vi "Get Pin Access.vi"(4 "Signature Method":T1=enum."HMAC-SHA1", 5 "Consumer Secret":string, 6 "Use External Browser? (F)":bool, 7 "Consumer Key":string, 8 "error in (no error)":errorcluster, 9 "Access URL":string, 10 "Authorize URL":string, 11 "Request URL":string) -> (0 "error out":errorcluster, 1 "OAuth Credentials":T2={"Consumer Key"="", "Signature Method"=enum."HMAC-SHA1", "Token"="", "Version"="", "Token Secret"="", "Consumer Secret"=""}, 2 "body":string, 3 "headers":string)   [LabVIEW 2011, in "i3-oauth.lvlib"]
doc: "Obtains OAuth Credentials via PIN authorization for the application specified by the <B>Consumer Key</B> and <B>Consumer Secret</B>"
uses:
  i3-oauth.lvlib
  Controls/OAuth Credentials.ctl
  Controls/Signature Method.ctl
panel:
  in  "Callback URL":string="oob"
  # "For pin access, the callback URL is always oob"
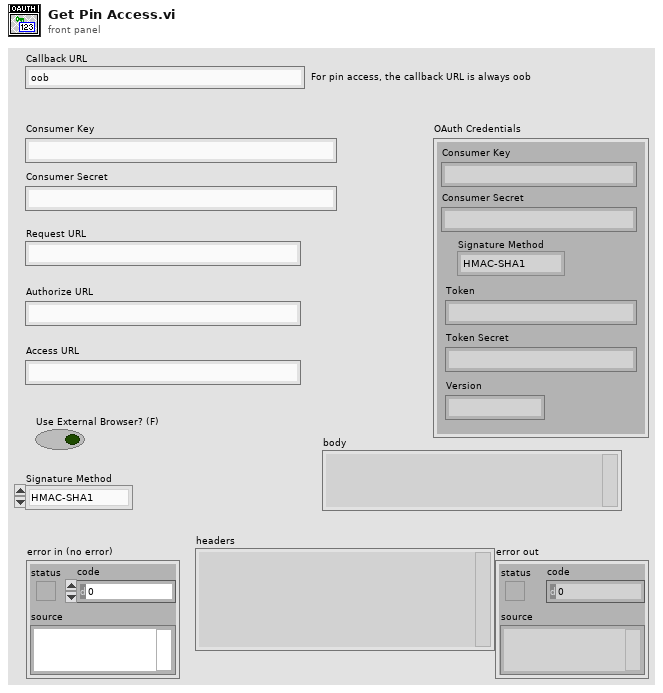
[diagram p1: front panel]
types:
  T1 = typedef "i3-oauth.lvlib/Signature Method.ctl" = enum16{"HMAC-MD5", "HMAC-SHA1", "HMAC-SHA224", "HMAC-SHA256", "HMAC-SHA384", "HMAC-SHA512"}
  T2 = typedef "i3-oauth.lvlib/OAuth Credentials.ctl" = cluster{"Consumer Key":string, "Signature Method":T1, "Token":string, "Version":string, "Token Secret":string, "Consumer Secret":string}
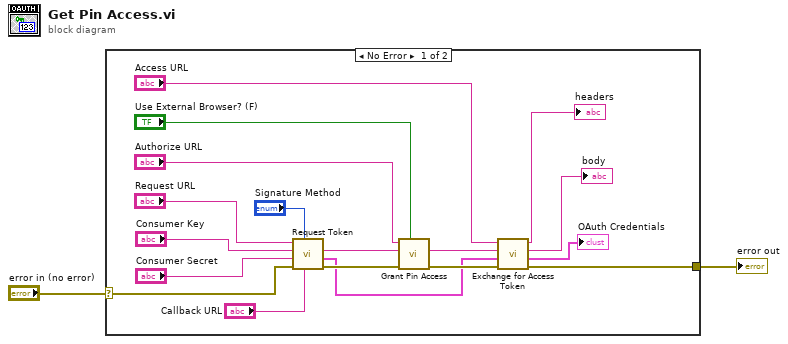
[diagram p0: block diagram]
diagram:
  n1 = case shown="No Error" "error in (no error)" {
    selector: "error in (no error)" -> [w11 w21]
    tunnel: [w10 w21] -> w1
    frame No Error {
      n2 = call "Request Token.vi"("Callback URL"="Callback URL", "Signature Method"="Signature Method", "error in (no error)"=w11, "Consumer Secret"="Consumer Secret", "Consumer Key"="Consumer Key", "Request URL"="Request URL") -> ("error out"=w20:errorcluster, "OAuth Credentials (request)"=w14:T2, "Request Token (duplicate)"=w13:string)  [unwired: 3 in]
      n3 = call "Grant Pin Access.vi"("Use External Browser? (F)"="Use External Browser? (F)", "error in (no error)"=w20, "Request token"=w13, "Authorize URL"="Authorize URL") -> ("error out"=w17:errorcluster, "Pin"=w15:string)  [unwired: 5 in, 1 out]
      n4 = call "Exchange for Access Token.vi"("error in (no error)"=w17, "OAuth Credentials (request)"=w14, "Pin"=w15, "Access Request URL"="Access URL") -> ("error out"=w10:errorcluster, "OAuth Credentials (access)"=→"OAuth Credentials":T2, "body"=→"body":string, "headers"=→"headers":string)  [unwired: 4 in]
    }
    frame Error {
    }
  }
  "error out" <- w1
